vi "SMTP Email [MAIL].vi"(4 "error in (no error)":errorcluster, 6 "return address":string, 7 "smtp session":T1) -> (0 "error out":errorcluster, 1 "reply":string, 2 "reply code":i32, 3 "smtp session out":T1)   [LabVIEW 2011, in "NewNI_SMTPEmail.lvlib"]
doc: "Sends the MAIL command to the SMTP server though connection specified as \"SMTP Session\", receives reply and interprets it. \n\nUser's e-mail is a desired return address.\n\nThis VI returns \"SMTP Session out,\" and the results of the error interpretation to the \"error out\" cluster."
uses:
  NewNI_SMTPEmail.lvlib
  SMTP Email Session.ctl
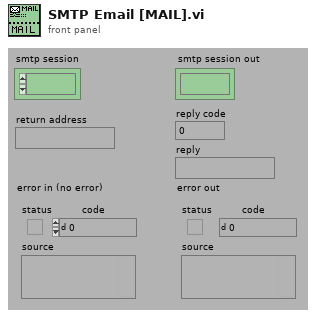
[diagram p1: front panel]
types:
  T1 = typedef "NewNI_SMTPEmail.lvlib/SMTP Email Session.ctl" = refnum<k1>
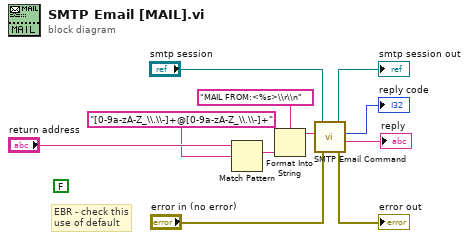
[diagram p0: block diagram]
diagram:
  (unwired) FALSE
  # "EBR - check this\nuse of default"
  n1 = Match Pattern(string="return address", regular expression="[0-9a-zA-Z_\\.\\-]+@[0-9a-zA-Z_\\.\\-]+") -> (match substring=w1:string)  [unwired: 4 out]
  n2 = Format Into String(format string="MAIL FROM:<%s>\\r\\n", w1) -> (resulting string=w7:string)  [unwired: 2 in, 1 out]
  n3 = call "SMTP Email Command.vi"("error in (no error)"="error in (no error)", "command"=w7, "smtp session"="smtp session") -> ("error out"=→"error out":errorcluster, "reply"=→"reply":string, "reply code"=→"reply code":i32, "smtp session out"=→"smtp session out":T1)  [unwired: 1 in]
